vi "MAIN.vi"() -> ()   [LabVIEW 2017]
uses:
  <vilib>/platform/TimedLoop/XDataNode/XDataNode.xnode
  <vilib>/Platform/TimedLoop/XDataNode/nitl_modes.ctl
  <vilib>/Platform/TimedLoop/XDataNode/XDNodeRunTimeDep.lvlib
  <vilib>/Platform/TimedLoop/XDataNode/wakeup.ctl
  <vilib>/Platform/TimedLoop/XDataNode/timing_clust.ctl
  GLOBALS.vi
panel:
  in  "Period 3":i64=20
  in  "Period 2":i64=20
  in  "Tab Control":enum32{"Page 1", "Page 2"}(tab)
  out "output cluster 4":cluster{"Média":dbl, "Variancia":dbl}
  out "output cluster 3":cluster{"Média":dbl, "Variancia":dbl}
  out "output cluster 2":cluster{"Média":dbl, "Variancia":dbl}
  out "output cluster":cluster{"Média":dbl, "Variancia":dbl}
  out "Chaveado":cluster{"x":dbl[], "Normal curve":dbl[]}(graph)
  out "Kalman":cluster{"x":dbl[], "Normal curve":dbl[]}(graph)
  out "Termico":cluster{"x":dbl[], "Normal curve":dbl[]}(graph)
  out "Pitot":cluster{"x":dbl[], "Normal curve":dbl[]}(graph)
  out "Pitot? 2":bool
  out "Térmico?":bool
  out "Pitot?":bool
  out "Kalman?":bool
  out "Chaveamento":dbl(graph)
  out "TERMICO":dbl(graph)
  out "PITOT":dbl(graph)
  in  "TERMICO Noise Amplitude 2":dbl=1.0
  out "KALMAN FUSED":dbl(graph)
  in  "PITOT Noise Amplitude 1":dbl=5.0
  in  "Input":dbl(slide) min=0.0 max=100.0 step=0.1 scale=0.0..100.0
  out "error":errorcluster
  in  "M":dbl=10.0
  out "Térmico?":bool
  in  "hmin":dbl=15.0
  in  "hmax":dbl=20.0
  in  "stop":bool
  in  "max":dbl=100.0
  in  "min":dbl
  # "Distribuições Normais"
  # "Medidas Puras"
  # "Medidas Fundidas"
  # "min e max eixo x"
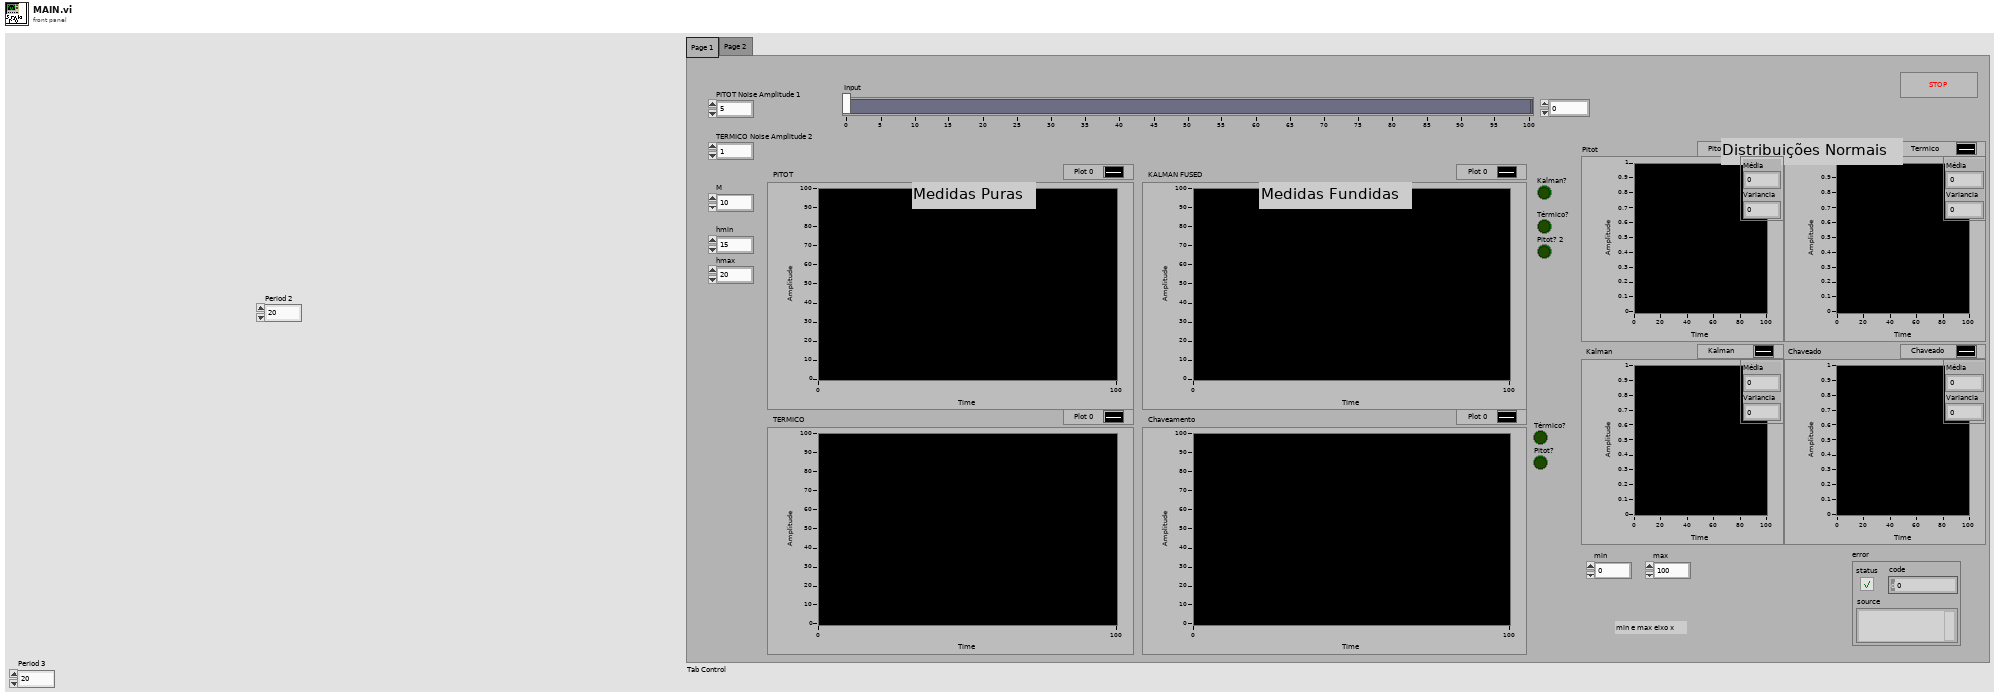
[diagram p1: front panel]
types:
  T1 = typedef "XDNodeRunTimeDep.lvlib/timing_clust.ctl" = cluster{"Expected End [f-1]":u64, "Actual End [f-1]":u64, "Finished Late? [f-1]":bool, "Expected End [i-1]":u64, "Actual End [i-1]":u64, "Finished Late? [i-1]":bool, "Expected Start [i]":u64, "Actual Start [i]":u64, "Expected Start [f]":u64, "Actual Start [f]":u64, "Source Name":string, "Structure Name":string, "Period":i64, "Deadline":i64, "Offset":i64, "Start":i64, "Priority":i32, "Timeout":i32, "Mode":T2, "Wakeup Reason":T3, "Error":errorcluster, "Source Type":string, "Secondary Source Type":string, "Global End Time":u64, "Global Start Time":u64, "Frame Duration":u64, "Iteration Duration":u64, "Assigned CPU":i32, "I/O Scan Engine Mode":u32}
  T2 = typedef "XDNodeRunTimeDep.lvlib/nitl_modes.ctl" = enum32{"No Change", "Process missed periods, maintain original phase", "Discard missed periods, maintain original phase", "Process missed periods, ignore original phase", "Discard missed periods, ignore original phase"}
  T3 = typedef "XDNodeRunTimeDep.lvlib/wakeup.ctl" = enum32{"Normal", "Aborted", "Asynchronous wakeup", "Timing source error", "Timed loop error", "Timeout"}
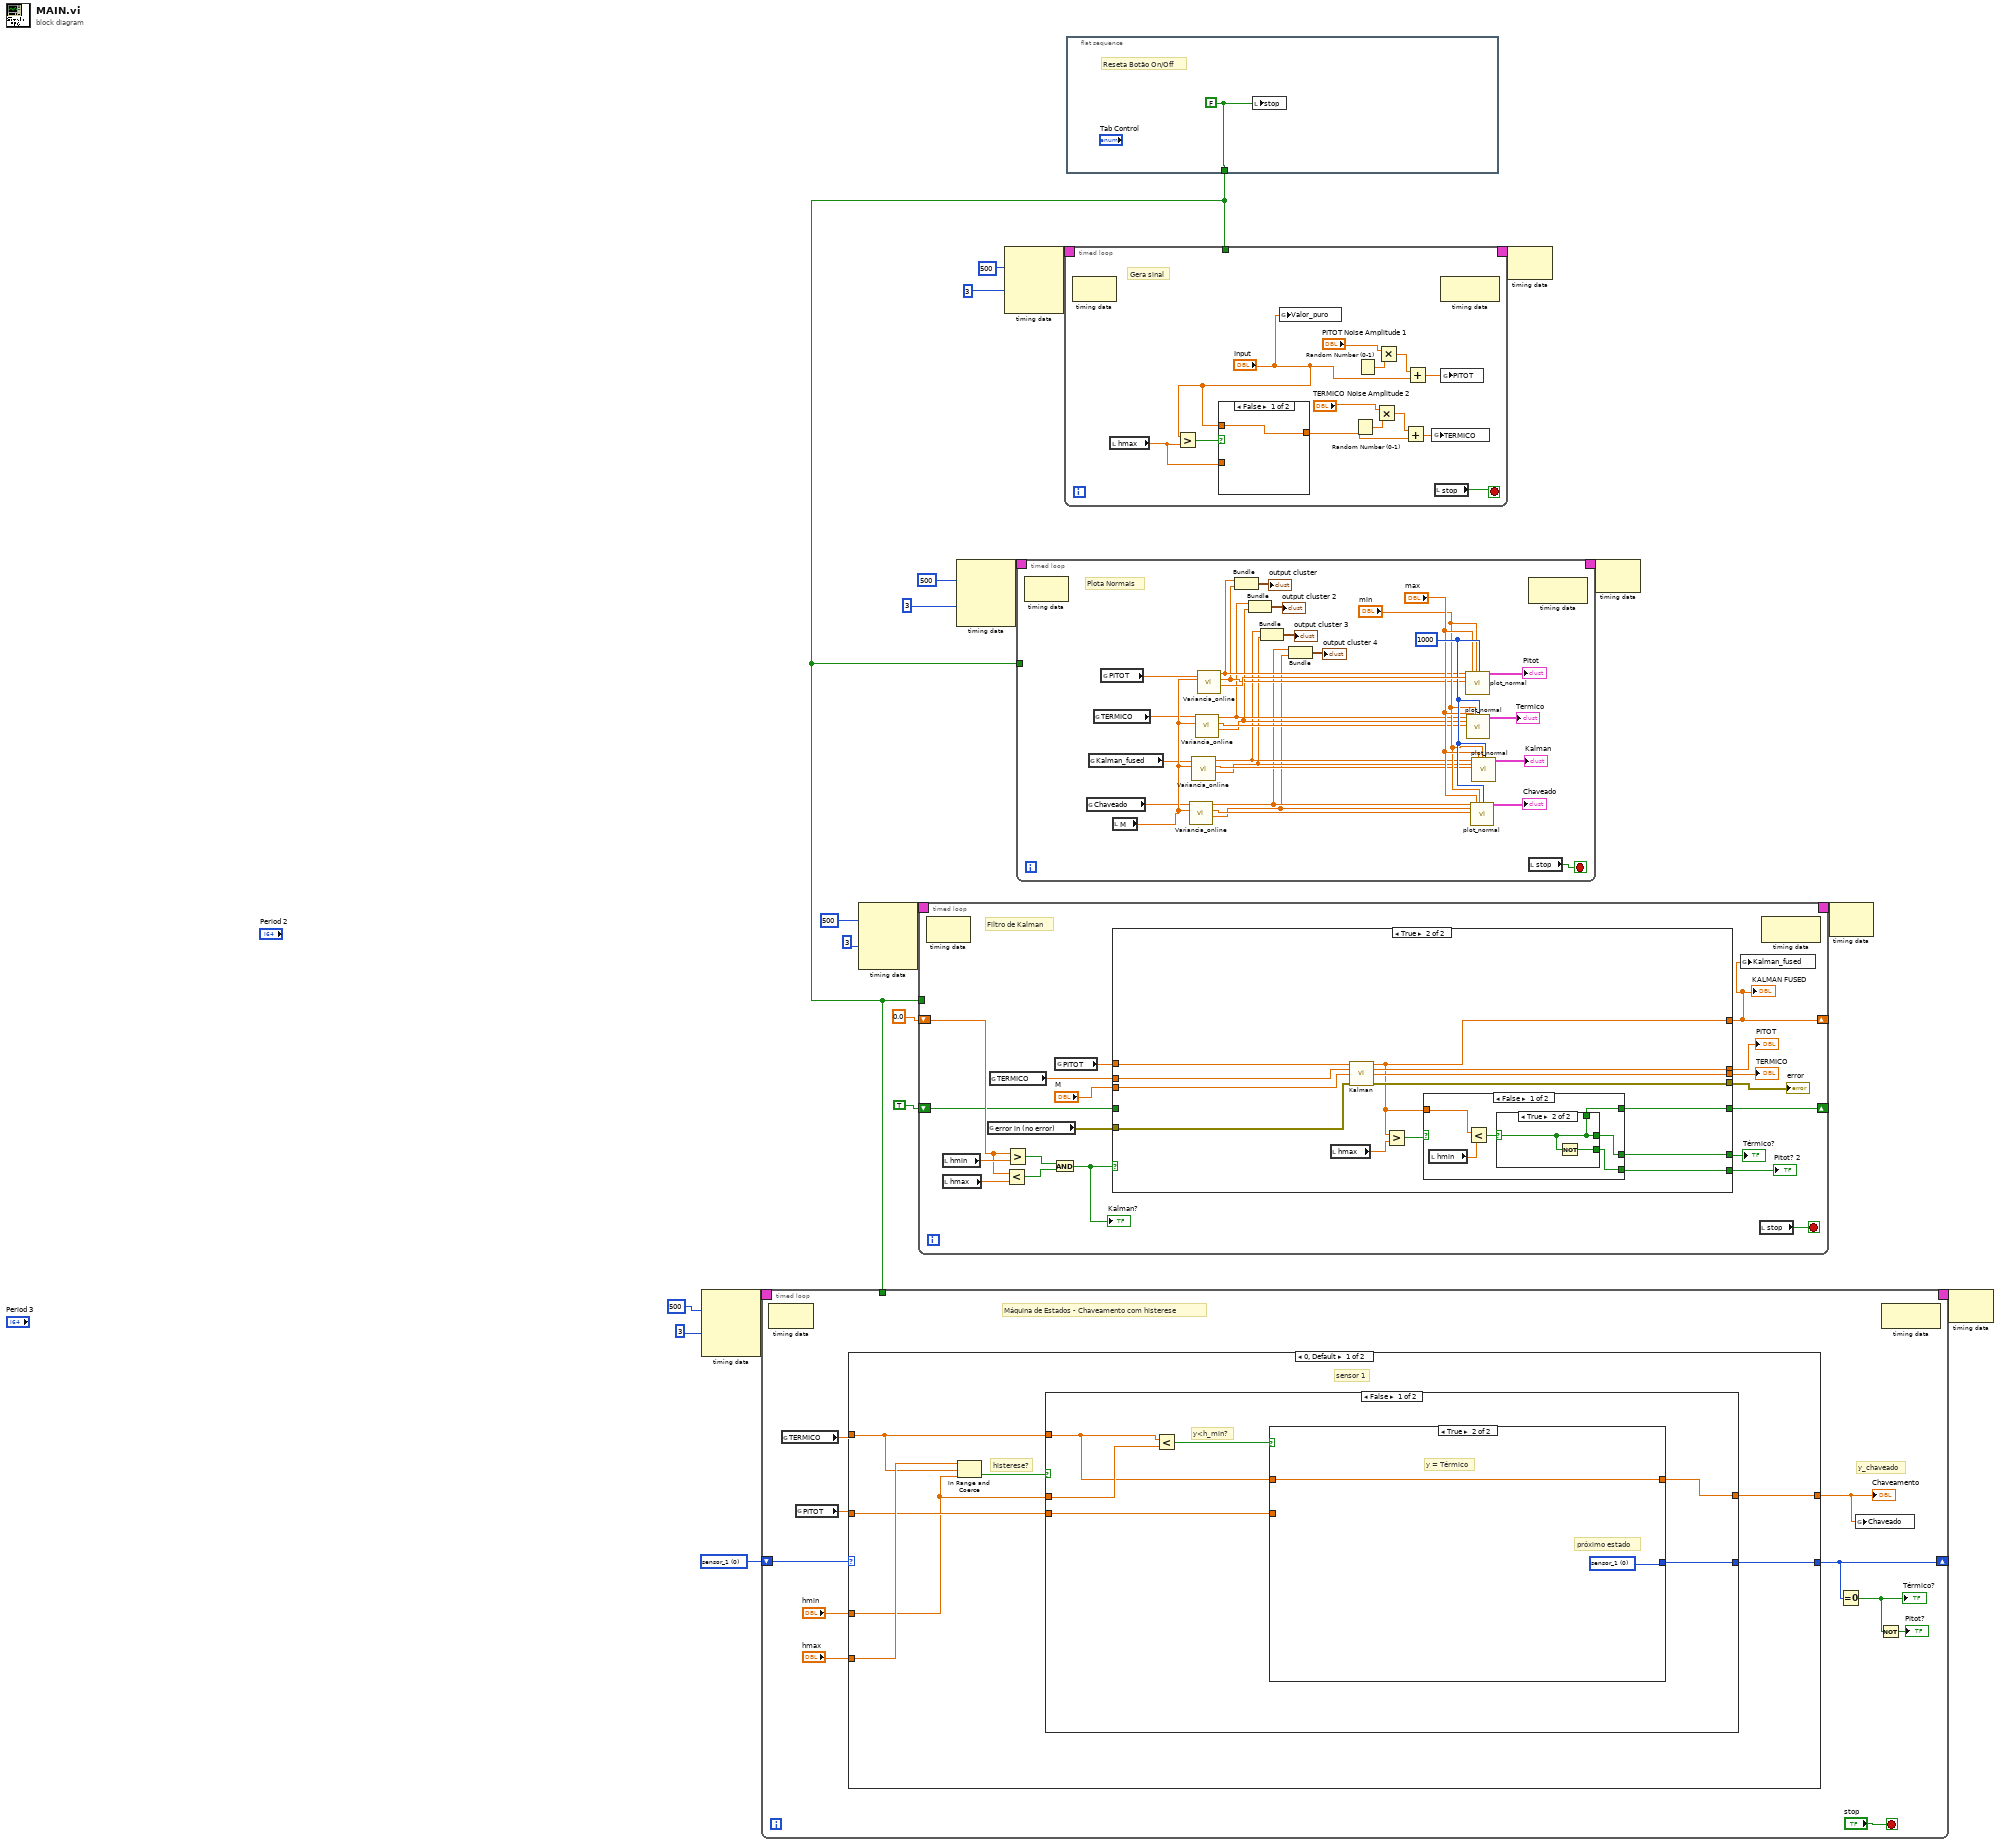
[diagram p0: block diagram]
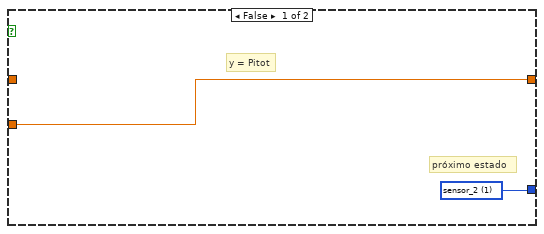
[diagram p2: hidden frame]
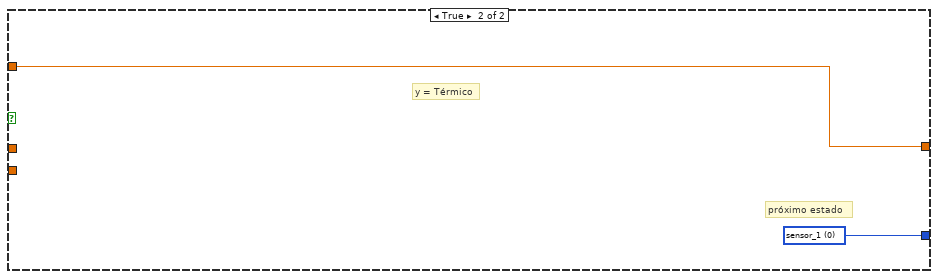
[diagram p3: hidden frame]
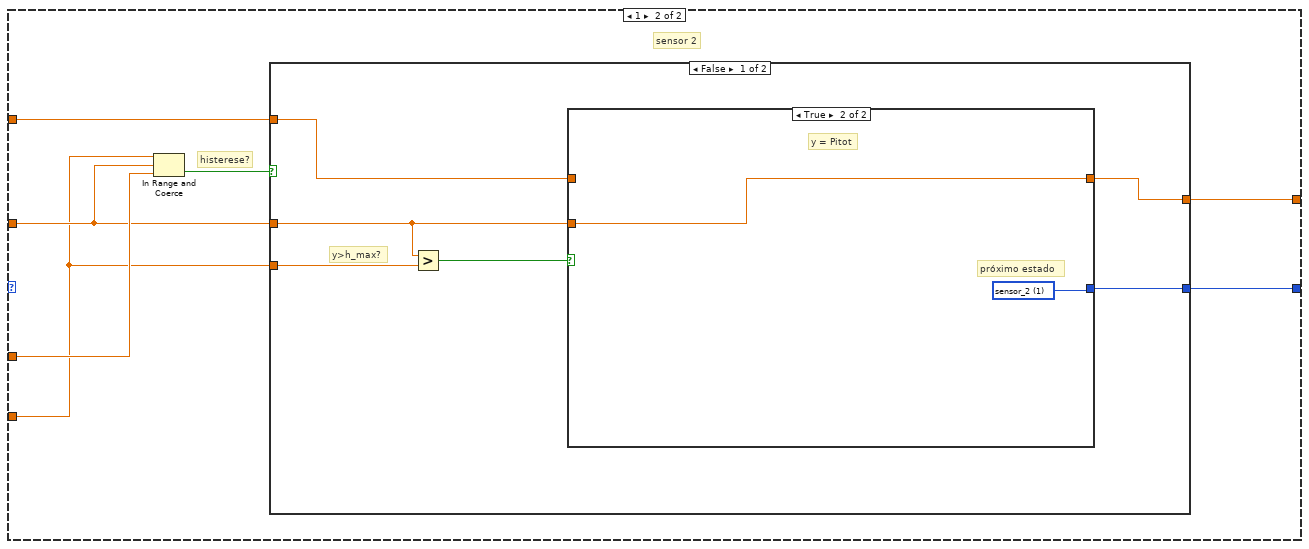
[diagram p4: hidden frame]
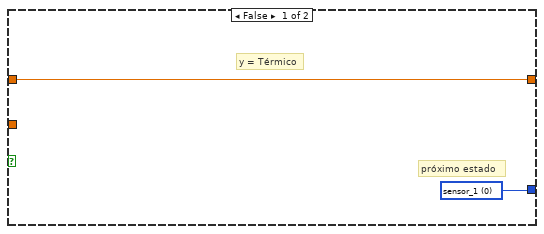
[diagram p5: hidden frame]
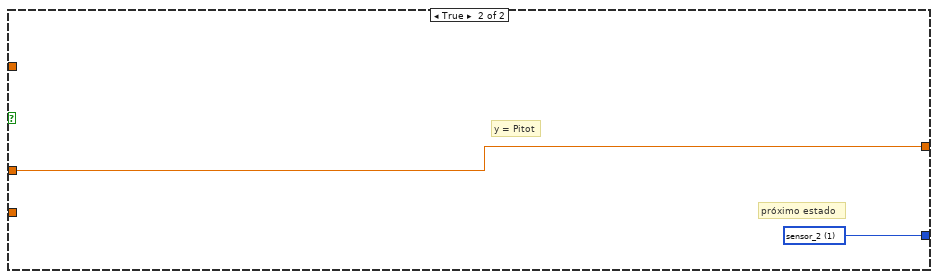
[diagram p6: hidden frame]
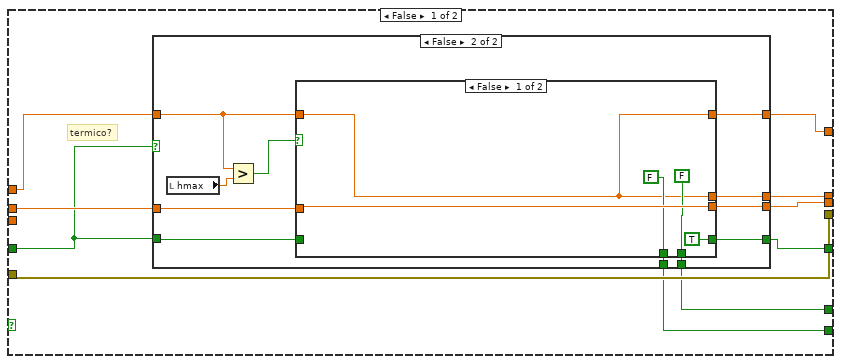
[diagram p7: hidden frame]
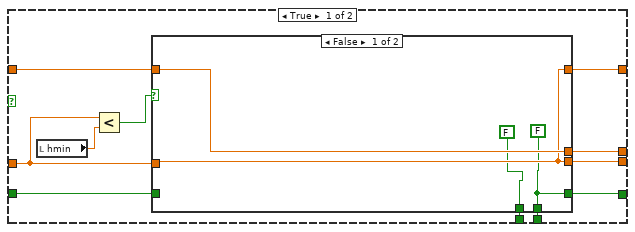
[diagram p8: hidden frame]
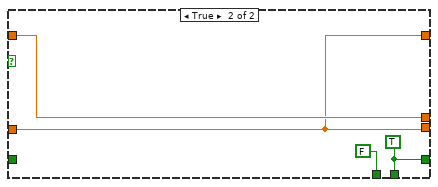
[diagram p9: hidden frame]
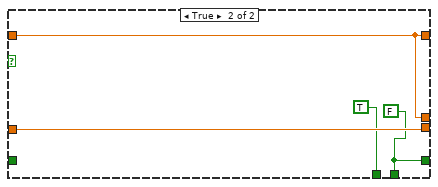
[diagram p10: hidden frame]
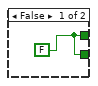
[diagram p11: hidden frame]
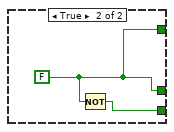
[diagram p12: hidden frame]
diagram:
  w12 = u16 0 items=["sensor_1", "sensor_2"] ("Sensor_inicial")
  n1 = node-c288(500 ("Priority"), 3 ("Priority")) -> (w14:T1)  [unwired: 2 in]
  n2 = timed-loop {
    shift-right: [w24] -> _
    shift-left: w12 -> [w30]
    timing: w14 -> [_]
    timing-out: [_] -> w13
    tunnel: w6 -> [_]
    stop <- "stop" stop-if-true
    # "Máquina de Estados - Chaveamento com histerese"
    # "y_chaveado"
    n3 = node-c288() -> ()  [unwired: 1 in, 1 out]
    n4 = global read "GLOBALS.vi" "TERMICO"() -> (w25:dbl)
    n5 = global read "GLOBALS.vi" "PITOT"() -> (w26:dbl)
    n6 = case shown="0, Default" w30 {
      tunnel: "hmin" -> [w33 w54]
      tunnel: "hmax" -> [w39 w52]
      tunnel: w25 -> [w36 w56]
      tunnel: w26 -> [w35 w53]
      tunnel: [w37 w57] -> w24
      tunnel: [w34 w55] -> w21
      frame 0, Default {
        # "histerese?"
        # "sensor 1"
        n7 = In Range and Coerce(upper limit=w39, x=w36, lower limit=w33) -> (In Range?=w38:bool)  [unwired: 1 out]
        n8 = case shown="False" w38 {
          tunnel: [w40 w51] -> w37
          tunnel: w36 -> [w43 w50]
          tunnel: w35 -> [w42 _]
          tunnel: [w41 w50] -> w34
          tunnel: w33 -> [w45 _]
          frame False {
            # "y<h_min?"
            n9 = Less?(x=w43, y=w45) -> (x < y?=w44:bool)
            n10 = case shown="True" w44 {
              tunnel: w43 -> [_ w49]
              tunnel: w42 -> [w47 _]
              tunnel: [w47 w49] -> w41
              tunnel: [w46 w48] -> w40
              frame False {
                w46 = u16 1 items=["sensor_1", "sensor_2"] ("Sensor_inicial")
                # "próximo estado"
                # "y = Pitot"
              }
              frame True {
                w48 = u16 0 items=["sensor_1", "sensor_2"] ("Sensor_inicial")
                # "próximo estado"
                # "y = Térmico"
              }
            }
          }
          frame True {
            w51 = u16 0 items=["sensor_1", "sensor_2"] ("Sensor_inicial")
            # "próximo estado"
            # "y = Térmico"
          }
        }
      }
      frame 1 {
        # "histerese?"
        # "sensor 2"
        n11 = In Range and Coerce(upper limit=w52, x=w53, lower limit=w54) -> (In Range?=w58:bool)  [unwired: 1 out]
        n12 = case shown="False" w58 {
          tunnel: [w60 w70] -> w57
          tunnel: w56 -> [w62 _]
          tunnel: w53 -> [w59 w69]
          tunnel: [w61 w69] -> w55
          tunnel: w52 -> [w64 _]
          frame False {
            # "y>h_max?"
            n13 = Greater?(x=w59, y=w64) -> (0:w63:bool)
            n14 = case shown="True" w63 {
              tunnel: w62 -> [w65 _]
              tunnel: w59 -> [_ w67]
              tunnel: [w65 w67] -> w61
              tunnel: [w66 w68] -> w60
              frame False {
                w66 = u16 0 items=["sensor_1", "sensor_2"] ("Sensor_inicial")
                # "próximo estado"
                # "y = Térmico"
              }
              frame True {
                w68 = u16 1 items=["sensor_1", "sensor_2"] ("Sensor_inicial")
                # "próximo estado"
                # "y = Pitot"
              }
            }
          }
          frame True {
            w70 = u16 1 items=["sensor_1", "sensor_2"] ("Sensor_inicial")
            # "próximo estado"
            # "y = Pitot"
          }
        }
      }
    }
    "Chaveamento" <- w21
    n15 = Equal To 0?(x=w24) -> (x = 0?=w22:bool)
    "Térmico?" <- w22
    n16 = global write "GLOBALS.vi" "Chaveado"(w21) -> ()
    n17 = Not(x=w22) -> (.not. x?=→"Pitot?":bool)
    n18 = node-c288() -> ()  [unwired: 1 in, 1 out]
  }
  n19 = node-c288(500 ("Priority"), 3 ("Priority")) -> (w17:T1)  [unwired: 2 in]
  n20 = timed-loop {
    timing: w17 -> [_]
    timing-out: [_] -> w16
    tunnel: w6 -> [_]
    shift-right: [w71] -> _
    shift-left: 0.0 ("y_fused") -> [w76]
    shift-right: [w73] -> _
    shift-left: TRUE -> [w72]
    stop <- w77 stop-if-true
    # "Filtro de Kalman"
    n21 = node-c288() -> ()  [unwired: 1 in, 1 out]
    n22 = local read "hmin"() -> (w83:dbl)
    n23 = local read "hmax"() -> (w82:dbl)
    n24 = global read "GLOBALS.vi" "error in (no error)"() -> (w89:errorcluster)
    n25 = global read "GLOBALS.vi" "TERMICO"() -> (w85:dbl)
    n26 = Less?(x=w76, y=w82) -> (x < y?=w80:bool)
    n27 = Greater?(x=w76, y=w83) -> (0:w81:bool)
    n28 = And(x=w81, y=w80) -> (x .and. y?=w78:bool)
    "Kalman?" <- w78
    n29 = global read "GLOBALS.vi" "PITOT"() -> (w86:dbl)
    n30 = case shown="True" w78 {
      tunnel: w89 -> [w99 w151]
      tunnel: "M" -> [_ w150]
      tunnel: [w99 w149] -> w87
      tunnel: [w98 w142] -> w71
      tunnel: w86 -> [w97 w148]
      tunnel: w85 -> [w95 w147]
      tunnel: [w96 w146] -> w79
      tunnel: [w94 w145] -> w84
      tunnel: [w93 w139] -> w75
      tunnel: [w92 w140] -> w74
      tunnel: [w91 w141] -> w73
      tunnel: w72 -> [w90 _]
      frame False {
        # "termico?"
        n31 = case shown="False" w90 {
          tunnel: [w110 w129] -> w98
          tunnel: w97 -> [w109 w123]
          tunnel: [w108 w128] -> w96
          tunnel: w95 -> [w104 w127]
          tunnel: [w107 w126] -> w94
          tunnel: [w106 w125] -> w93
          tunnel: [w105 w124] -> w92
          tunnel: [w101 w120] -> w91
          tunnel: w90 -> [w100 w119]
          frame True {
            n32 = local read "hmin"() -> (w103:dbl)
            n33 = Less?(x=w104, y=w103) -> (x < y?=w102:bool)
            n34 = case shown="False" w102 {
              tunnel: [w113 w117] -> w110
              tunnel: w109 -> [w114 w118]
              tunnel: [w114 w118] -> w108
              tunnel: [w113 w117] -> w107
              tunnel: w104 -> [w113 w117]
              tunnel: [FALSE FALSE] -> w106
              tunnel: [w111 w115] -> w105
              tunnel: [w111 w115] -> w101
              tunnel: w100 -> [_ _]
              frame False {
                w111 = FALSE
              }
              frame True {
                w115 = TRUE
              }
            }
          }
          frame False {
            n35 = local read "hmax"() -> (w122:dbl)
            n36 = Greater?(x=w123, y=w122) -> (0:w121:bool)
            n37 = case shown="False" w121 {
              tunnel: [w131 w137] -> w129
              tunnel: w123 -> [w131 w137]
              tunnel: [w131 w137] -> w128
              tunnel: [w134 w138] -> w126
              tunnel: w127 -> [w134 w138]
              tunnel: [FALSE TRUE] -> w125
              tunnel: [FALSE w135] -> w124
              tunnel: [TRUE w135] -> w120
              tunnel: w119 -> [_ _]
              frame False {
              }
              frame True {
                w135 = FALSE
              }
            }
          }
        }
      }
      frame True {
        n38 = local read "hmax"() -> (w144:dbl)
        n39 = call "Kalman.vi"("y1"=w148, "y2"=w147, "M"=w150, "error in (no error)"=w151) -> ("y_fused"=w142:dbl, "y1"=w146:dbl, "y2"=w145:dbl, "error out"=w149:errorcluster)  [unwired: 6 in, 2 out]
        n40 = Greater?(x=w142, y=w144) -> (0:w143:bool)
        n41 = case shown="False" w143 {
          tunnel: w142 -> [w156 _]
          tunnel: [w154 w161] -> w141
          tunnel: [w153 w161] -> w140
          tunnel: [w152 w162] -> w139
          frame False {
            n42 = local read "hmin"() -> (w155:dbl)
            n43 = Less?(x=w156, y=w155) -> (x < y?=w157:bool)
            n44 = case shown="True" w157 {
              selector: w157 -> [_ w159]
              tunnel: [_ w159] -> w154
              tunnel: [w158 w159] -> w153
              tunnel: [w158 w160] -> w152
              frame False {
                w158 = FALSE
              }
              frame True {
                n45 = Not(x=w159) -> (.not. x?=w160:bool)
              }
            }
          }
          frame True {
            w161 = FALSE
            n46 = Not(x=w161) -> (.not. x?=w162:bool)
          }
        }
      }
    }
    "error" <- w87
    "KALMAN FUSED" <- w71
    "PITOT" <- w79
    "TERMICO" <- w84
    "Térmico?" <- w74
    "Pitot? 2" <- w75
    n47 = global write "GLOBALS.vi" "Kalman_fused"(w71) -> ()
    n48 = local read "stop"() -> (w77:bool)
    n49 = node-c288() -> ()  [unwired: 1 in, 1 out]
  }
  n50 = node-c288(500 ("Priority"), 3 ("Priority")) -> (w8:T1)  [unwired: 2 in]
  n51 = node-c288(500 ("Priority"), 3 ("Priority")) -> (w20:T1)  [unwired: 2 in]
  n52 = timed-loop {
    timing: w8 -> [_]
    timing-out: [_] -> w7
    tunnel: w6 -> [_]
    stop <- w193 stop-if-true
    w186 = u16 1000 ("N")
    # "Plota Normais"
    n53 = node-c288() -> ()  [unwired: 1 in, 1 out]
    n54 = global read "GLOBALS.vi" "Chaveado"() -> (w188:dbl)
    n55 = global read "GLOBALS.vi" "Kalman_fused"() -> (w189:dbl)
    n56 = global read "GLOBALS.vi" "TERMICO"() -> (w190:dbl)
    n57 = global read "GLOBALS.vi" "PITOT"() -> (w191:dbl)
    n58 = local read "M"() -> (w192:dbl)
    n59 = call "Variancia_online.vi"("M"=w192, "u"=w188) -> ("std"=w165:dbl, "var"=w183:dbl, "y"=w166:dbl)  [unwired: 6 in, 1 out]
    n60 = call "Variancia_online.vi"("M"=w192, "u"=w189) -> ("std"=w167:dbl, "var"=w182:dbl, "y"=w168:dbl)  [unwired: 6 in, 1 out]
    n61 = call "Variancia_online.vi"("M"=w192, "u"=w190) -> ("std"=w169:dbl, "var"=w181:dbl, "y"=w170:dbl)  [unwired: 6 in, 1 out]
    n62 = call "Variancia_online.vi"("M"=w192, "u"=w191) -> ("std"=w187:dbl, "var"=w175:dbl, "y"=w176:dbl)  [unwired: 6 in, 1 out]
    n63 = Bundle("y"=w176, "var"=w175) -> (→"output cluster":cluster{"y":dbl, "var":dbl})  [unwired: 1 in]
    n64 = Bundle("y"=w170, "std"=w169) -> (→"output cluster 2":cluster{"y":dbl, "std":dbl})  [unwired: 1 in]
    n65 = Bundle("y"=w168, "std"=w167) -> (→"output cluster 3":cluster{"y":dbl, "std":dbl})  [unwired: 1 in]
    n66 = Bundle("y"=w166, "std"=w165) -> (→"output cluster 4":cluster{"y":dbl, "std":dbl})  [unwired: 1 in]
    n67 = call "plot_normal.vi"("mean"=w176, "standard deviation"=w187, "variance"=w175, "xsup"="max", "xinf"="min", "N"=w186) -> ("Normal_xy"=→"Pitot":cluster{dbl[], dbl[]})  [unwired: 10 in, 3 out]
    n68 = call "plot_normal.vi"("mean"=w170, "standard deviation"=w169, "variance"=w181, "xsup"="max", "xinf"="min", "N"=w186) -> ("Normal_xy"=→"Termico":cluster{dbl[], dbl[]})  [unwired: 10 in, 3 out]
    n69 = call "plot_normal.vi"("mean"=w166, "standard deviation"=w165, "variance"=w183, "xsup"="max", "xinf"="min", "N"=w186) -> ("Normal_xy"=→"Chaveado":cluster{dbl[], dbl[]})  [unwired: 10 in, 3 out]
    n70 = call "plot_normal.vi"("mean"=w168, "standard deviation"=w167, "variance"=w182, "xsup"="max", "xinf"="min", "N"=w186) -> ("Normal_xy"=→"Kalman":cluster{dbl[], dbl[]})  [unwired: 10 in, 3 out]
    n71 = node-c288() -> ()  [unwired: 1 in, 1 out]
    n72 = local read "stop"() -> (w193:bool)
  }
  n73 = timed-loop {
    timing: w20 -> [_]
    timing-out: [_] -> w19
    tunnel: w6 -> [_]
    stop <- w197 stop-if-true
    # "Gera sinal"
    n74 = node-c288() -> ()  [unwired: 1 in, 1 out]
    n75 = local read "hmax"() -> (w198:dbl)
    n76 = Greater?(x="Input", y=w198) -> (0:w200:bool)
    n77 = case shown="False" w200 {
      tunnel: w198 -> [_ w210]
      tunnel: [w209 w210] -> w199
      tunnel: "Input" -> [w209 _]
      frame False {
      }
      frame True {
      }
    }
    n78 = global write "GLOBALS.vi" "Valor_puro"("Input") -> ()
    n79 = Random Number (0-1)() -> (number: 0 to 1=w202:dbl)
    n80 = Random Number (0-1)() -> (number: 0 to 1=w208:dbl)
    n81 = Multiply(x="TERMICO Noise Amplitude 2", y=w202) -> (x*y=w203:dbl)
    n82 = Multiply(x="PITOT Noise Amplitude 1", y=w208) -> (x*y=w206:dbl)
    n83 = Add(x=w203, y=w199) -> (x+y=w204:dbl)
    n84 = Add(x=w206, y="Input") -> (x+y=w205:dbl)
    n85 = global write "GLOBALS.vi" "TERMICO"(w204) -> ()
    n86 = local read "stop"() -> (w197:bool)
    n87 = node-c288() -> ()  [unwired: 1 in, 1 out]
    n88 = global write "GLOBALS.vi" "PITOT"(w205) -> ()
  }
  n89 = flat-sequence {
    tunnel: [w213] -> w6
    frame #0 {
      w213 = FALSE ("stop")
      # "Reseta Botão On/Off"
      n90 = local write "stop"(w213) -> ()
    }
  }
  n91 = node-c288(w19) -> ()  [unwired: 1 out]
  n92 = node-c288(w7) -> ()  [unwired: 1 out]
  n93 = node-c288(w16) -> ()  [unwired: 1 out]
  n94 = node-c288(w13) -> ()  [unwired: 1 out]
